vi "Error Handle.vi"() -> ()   [LabVIEW 2016]
uses:
  <vilib>/Utility/error.llb/DialogType.ctl
  Architecture/Queue Management/ARC_Queue Create_Single.vi
  Architecture/Queue Management/ARC_Queue Valid.vi
  Architecture/Queue Management/ARC_Queue Insert Element.vi
  Architecture/Queue Management/ARC_Queue Remove Element.vi
  Architecture/Queue Management/ARC_Queue Destroy_Single.vi
panel:
  in  "Parameter":cluster{"Q-Local":string, "Variant":variant}
  out "Error Report":string
  out "Current State":string
  in  "Exit Program":bool
  in  "TempVariable":T1
  # "/* -------- Notes for All Users -------- */\nRecommand : \n[1].Display Setting Resolution -> 1440x900\n[2].Read Arch Notes First.\n[3].Make A Call When You Are In Trouble.\n\nTeam Members:\nPansino Soft,Pansino SDMA\n\nCopyright@2013 Pansino.Beijing\n\nVersion Number: 2013"
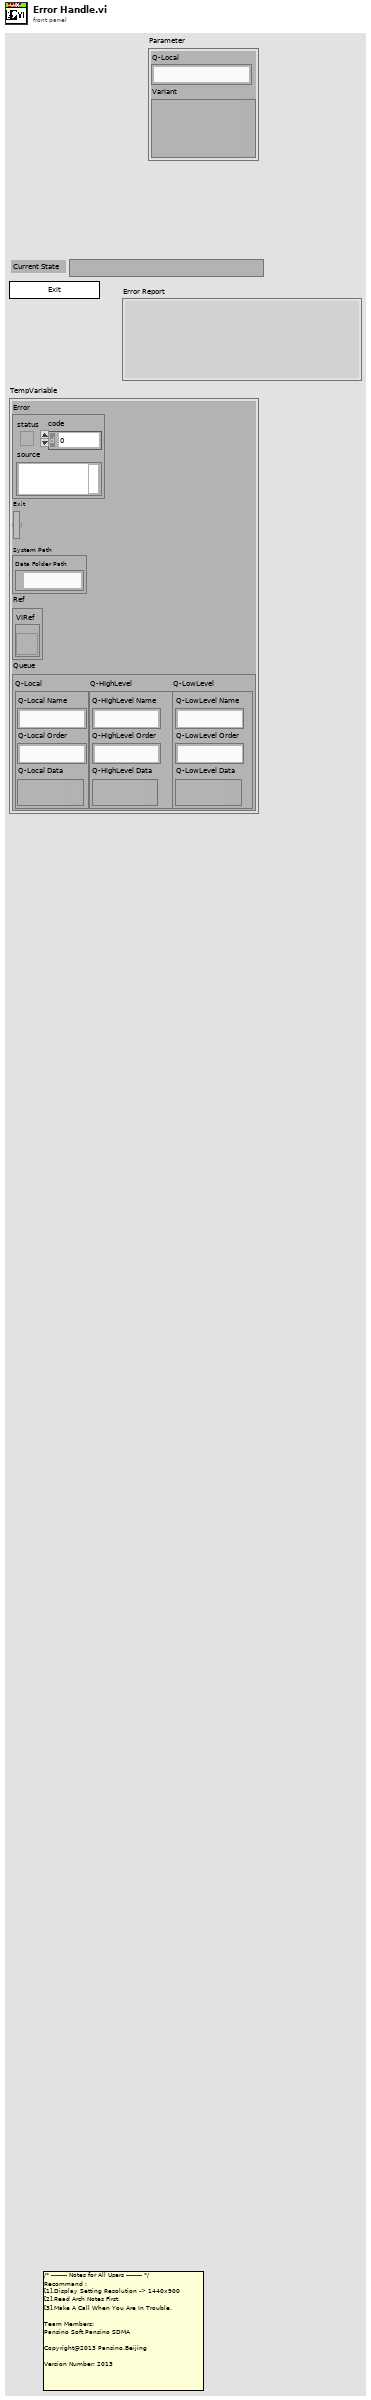
[diagram p1: front panel]
types:
  T1 = cluster{"Error":errorcluster, "Exit":bool, "System Path":cluster{"Data Folder Path":path}, "Ref":cluster{"VIRef":refnum<vi>}, "Queue":cluster{"Q-Local":cluster{"Q-Local Name":string, "Q-Local Order":string, "Q-Local Data":variant}, "Q-HighLevel":cluster{"Q-HighLevel Name":string, "Q-HighLevel Order":string, "Q-HighLevel Data":variant}, "Q-LowLevel":cluster{"Q-LowLevel Name":string, "Q-LowLevel Order":string, "Q-LowLevel Data":variant}}}
  T2 = typedef "DialogType.ctl" = u16
  T3 = cluster{"DfltDataFolder":path, "ParaFolder":path, "SysCfg":path, "CHdef":path, "ModCfg":path, "DT Folder":path, "ErrorLog":path, "HBMlic":path, "HBMDriver":path}
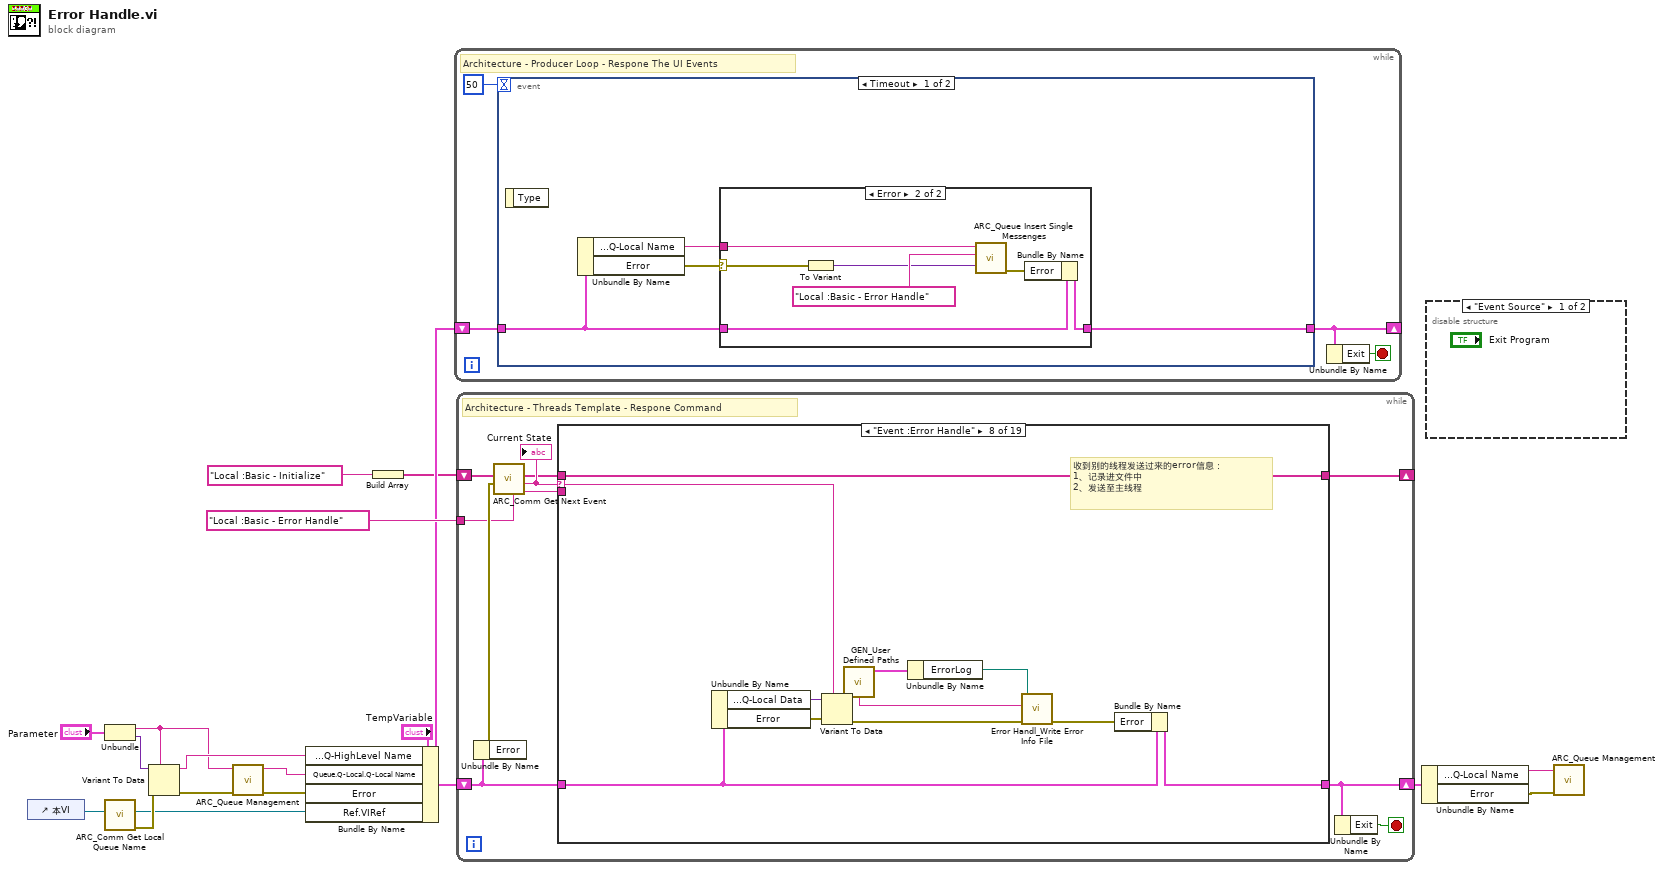
[diagram p0: block diagram]
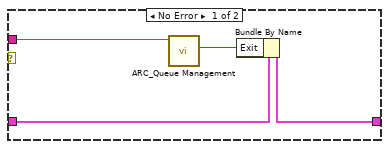
[diagram p2: hidden frame]
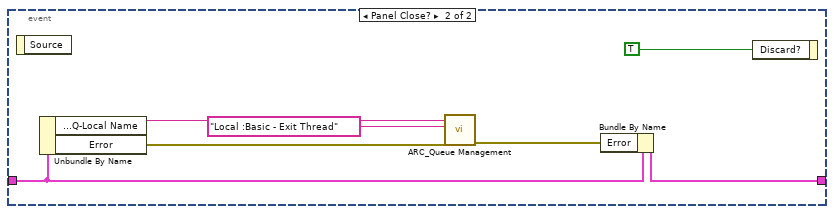
[diagram p3: hidden frame]
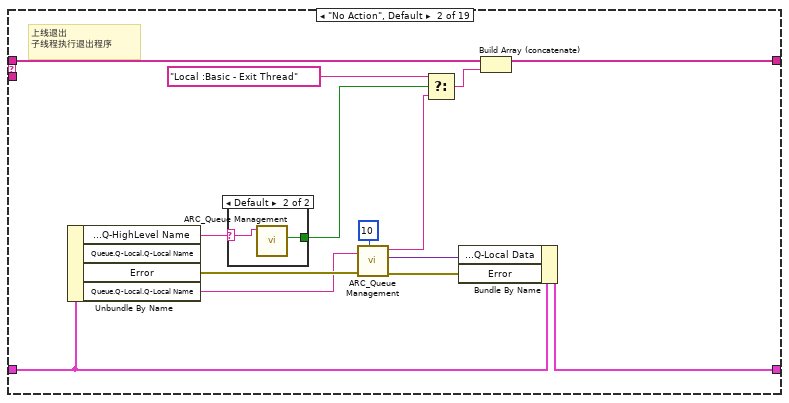
[diagram p6: hidden frame]
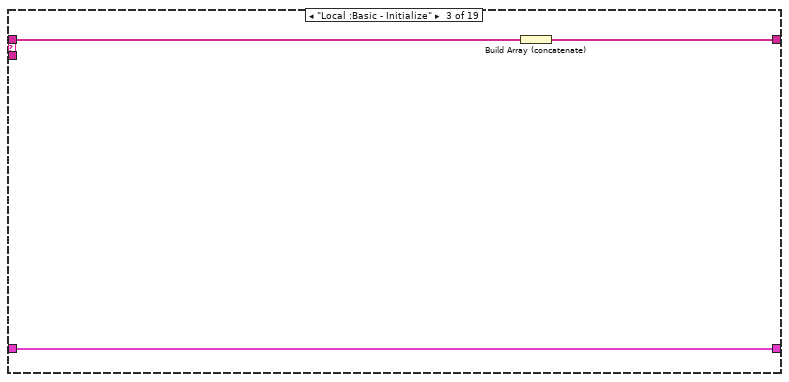
[diagram p8: hidden frame]
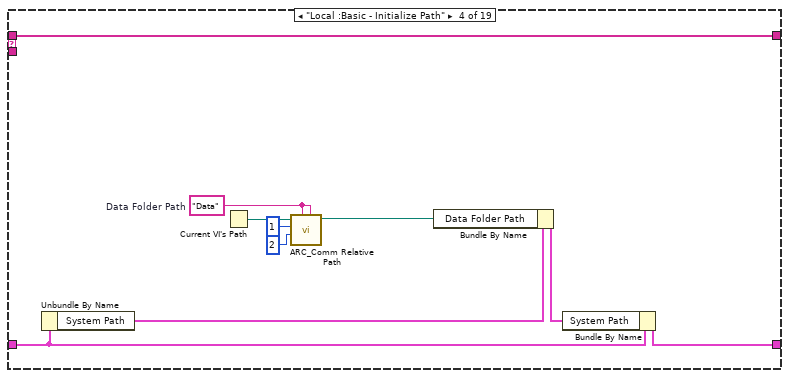
[diagram p9: hidden frame]
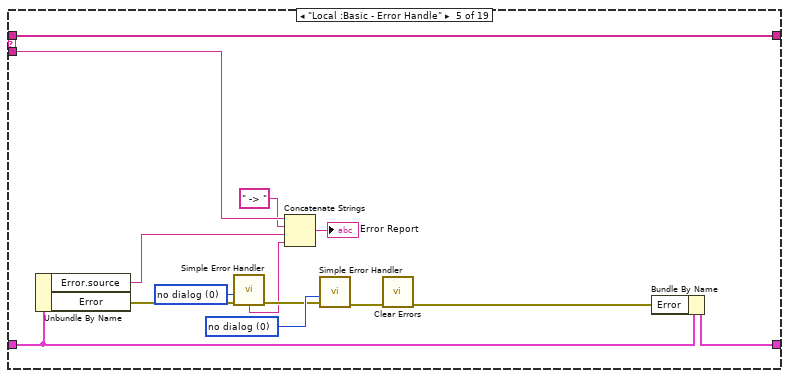
[diagram p10: hidden frame]
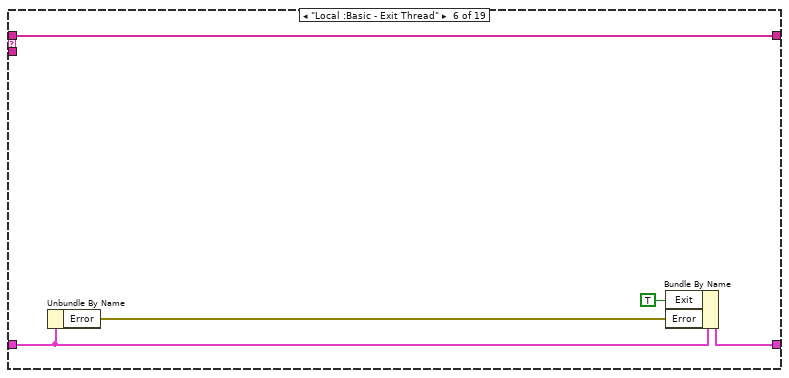
[diagram p11: hidden frame]
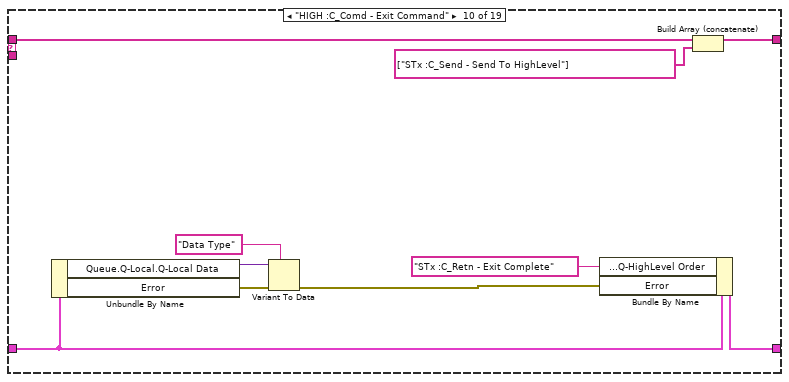
[diagram p14: hidden frame]
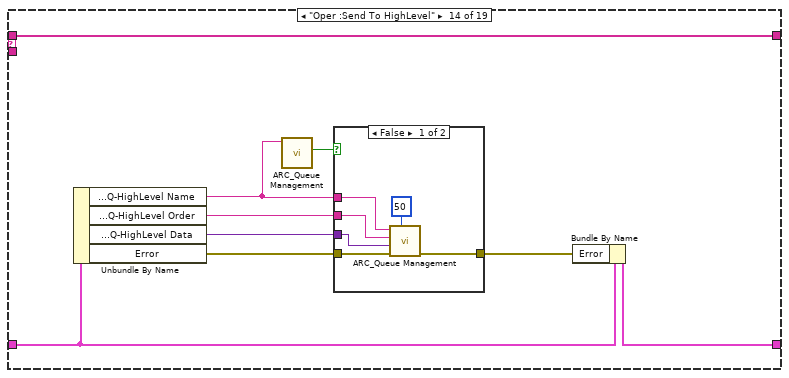
[diagram p18: hidden frame]
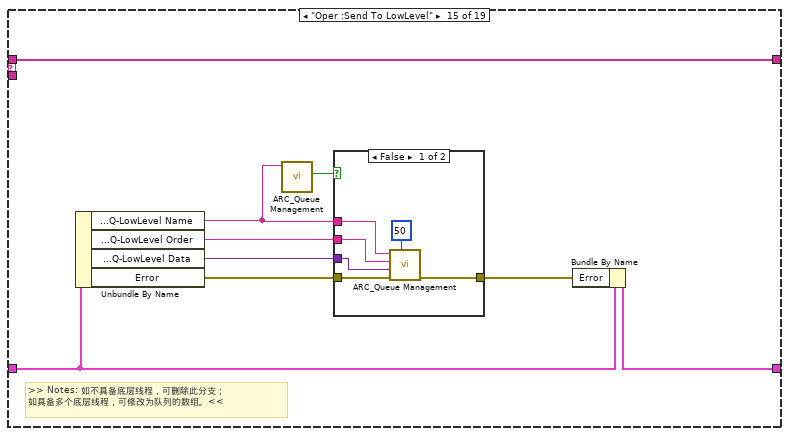
[diagram p20: hidden frame]
diagram:
  n1 = control-ref of="本VI"() -> (w7:refnum<vi>)
  n2 = Unbundle("Parameter") -> ("Q-Local"=w1:string, "Variant"=w10:variant)
  n3 = call "ARC_Comm Get Local Queue Name.vi"("VI Ref"=w7) -> ("error out"=w8:errorcluster, "VI Ref out"=w5:refnum<vi>)  [unwired: 8 in, 1 out]
  n4 = Variant To Data(error in=w8, type=w1, Variant=w10) -> (data=w2:string, error out=w6:errorcluster)
  n5 = call-poly "ARC_Queue Management.vi"("error in"=w6, "Queue Name"=w1) -> ("error out"=w4:errorcluster, "Queue Name dup"=w3:string)  [unwired: 7 in, 1 out]
  n6 = Bundle By Name(cluster="TempVariable", "Queue.Q-HighLevel.Q-HighLevel Name"=w2, "Queue.Q-Local.Q-Local Name"=w3, "Error"=w4, "Ref.VIRef"=w5) -> (w13:T1)
  n7 = Build Array("Local :Basic - Initialize") -> (w11:string[])
  n8 = while {
    shift-right: [w20] -> _
    shift-left: w13 -> [w21]
    stop <- w19 stop-if-true
    # "Architecture - Producer Loop - Respone The UI Events"
    n9 = event shown="[0] Timeout" {
      selector: _ -> [_ _]
      dyn-events: _ -> [_ _]
      timeout: 50 -> [_ _]
      tunnel: w21 -> [w25 w42]
      tunnel: [w26 w41] -> w20
      event Timeout {
        n10 = event-data() -> ()  [unwired: 1 in, 1 out]
        n11 = Unbundle By Name(w25) -> ("Queue.Q-Local.Q-Local Name"=w24:string, "Error"=w23:errorcluster)
        n12 = case shown="Error" w23 {
          selector: w23 -> [_ w37]
          tunnel: [w30 w35] -> w26
          tunnel: w25 -> [w28 w36]
          tunnel: w24 -> [w27 w34]
          frame No Error {
            n13 = call-poly "ARC_Queue Management.vi"("Queue Name(unamed)"=w27) -> ("Not Exist?"=w29:bool)  [unwired: 8 in, 2 out]
            n14 = Bundle By Name(cluster=w28, "Exit"=w29) -> (w30:T1)
          }
          frame Error {
            n15 = To Variant(anything=w37) -> (Variant=w32:variant)
            n16 = call "ARC_Queue Insert Single Messenges.vi"("Data"=w32, "Order"="Local :Basic - Error Handle" ("Event"), "Queue Name"=w34) -> ("error out"=w31:errorcluster)  [unwired: 8 in]
            n17 = Bundle By Name(cluster=w36, "Error"=w31) -> (w35:T1)
          }
        }
      }
      event Panel Close? {
        n18 = event-data() -> ()  [unwired: 1 in, 1 out]
        n19 = Unbundle By Name(w42) -> ("Queue.Q-Local.Q-Local Name"=w39:string, "Error"=w43:errorcluster)
        n20 = call-poly "ARC_Queue Management.vi"("error in (no error)"=w43, "Event"="Local :Basic - Exit Thread", "Queue Name(unamed)"=w39) -> ("error out"=w40:errorcluster)  [unwired: 7 in, 1 out]
        n21 = Bundle By Name(cluster=w42, "Error"=w40) -> (w41:T1)
        n22 = event-data("Discard?"=TRUE ("放弃？")) -> ()  [unwired: 1 in, 1 out]
      }
    }
    n23 = Unbundle By Name(w20) -> ("Exit"=w19:bool)
  }
  n24 = while {
    shift-right: [w48] -> w18
    shift-left: w13 -> [w50]
    shift-right: [w51] -> _
    shift-left: w11 -> [w54]
    tunnel: "Local :Basic - Error Handle" ("Error Handle") -> [w46]
    stop <- w47 stop-if-true
    # "Architecture - Threads Template - Respone Command"
    n25 = Unbundle By Name(w50) -> ("Error"=w49:errorcluster)
    n26 = call "ARC_Comm Get Next Event.vi"("Error Handle"=w46, "error in (no error)"=w49, "event queue in"=w54) -> ("prev event"=w45:string, "next event"=w53:string, "event queue out"=w52:string[])  [unwired: 3 in]
    "Current State" <- w53
    n27 = case shown="\"Event :Error Handle\"" w53 {
      selector: w53 -> [_ _ _ _ _ _ _ w113 _ _ _ _ _ _ _ _ _ _ _]
      tunnel: w50 -> [w55 w70 w74 w83 w97 w101 w105 w116 w118 w126 w130 w132 w134 w141 w157 w168 w173 w180 w186]
      tunnel: w52 -> [w56 w63 w75 w85 w99 w104 w106 w117 w119 w129 w131 w133 w135 w144 w160 w169 w171 w181 w184]
      tunnel: [w56 w62 w73 w85 w99 w104 w106 w117 w119 w127 w131 w133 w135 w144 w160 w169 w170 w181 w183] -> w51
      tunnel: [w55 w69 w74 w84 w98 w102 w105 w108 w118 w128 w130 w132 w134 w140 w156 w168 w172 w179 w185] -> w48
      tunnel: w45 -> [_ _ _ _ w90 _ _ _ _ _ _ _ _ _ _ _ _ _ _]
      frame "----------Core Status----------" {
      }
      frame "No Action", Default {
        # "上线退出\n子线程执行退出程序"
        n28 = Unbundle By Name(w70) -> ("Queue.Q-HighLevel.Q-HighLevel Name"=w65:string, "Error"=w66:errorcluster, "Queue.Q-Local.Q-Local Name"=w64:string)  [unwired: 1 out]
        n29 = case shown="Default" w65 {
          selector: w65 -> [_ w71]
          tunnel: [_ w72] -> w60
          frame "" {
          }
          frame Default {
            n30 = call-poly "ARC_Queue Management.vi"("Queue Name(unamed)"=w71) -> ("Not Exist?"=w72:bool)  [unwired: 8 in, 2 out]
          }
        }
        n31 = call-poly "ARC_Queue Management.vi"("Time out(-1)_queue out"=10, "error in (no error)"=w66, "Queue Name(unamed)"=w64) -> ("error out"=w68:errorcluster, "Data"=w67:variant, "Event"=w58:string)  [unwired: 5 in, 1 out]
        n32 = Select(t="Local :Basic - Exit Thread" ("Event"), s=w60, f=w58) -> (s? t:f=w57:string)
        n33 = Bundle By Name(cluster=w70, "Queue.Q-Local.Q-Local Data"=w67, "Error"=w68) -> (w69:T1)
        n34 = Build Array (concatenate)(w63, w57) -> (w62:string[])
      }
      frame "Local :Basic - Initialize" {
        n35 = Build Array (concatenate)(w75) -> (w73:string[])
      }
      frame "Local :Basic - Initialize Path" {
        w78 = "Data"  # Data Folder Path
        n36 = Unbundle By Name(w83) -> ("System Path"=w77:cluster{"Data Folder Path":path})
        n37 = Current VI's Path() -> (path=w79:path)
        n38 = call "ARC_Comm Relative Path.vi"("Development Relative Path"=w78, "Run Time relative path"=w78, "Run-Time File Depth"=2, "Development File Depth"=1, "Root Path"=w79) -> ("Relative Path"=w82:path)  [unwired: 5 in, 1 out]
        n39 = Bundle By Name(cluster=w77, "Data Folder Path"=w82) -> (w76:cluster{"Data Folder Path":path})
        n40 = Bundle By Name(cluster=w83, "System Path"=w76) -> (w84:T1)
      }
      frame "Local :Basic - Error Handle" {
        w91 = T2 0 items=["no dialog", "OK message", "continue or stop message", "OK message + warnings", "continue/stop + warnings"] ("type of dialog (OK msg:1)")
        w94 = T2 0 items=["no dialog", "OK message", "continue or stop message", "OK message + warnings", "continue/stop + warnings"] ("type of dialog (OK msg:1)")
        n41 = Unbundle By Name(w97) -> ("Error.source"=w86:string, "Error"=w93:errorcluster)
        n42 = call <vilib>:"Simple Error Handler.vi"("type of dialog (OK msg:1)"=w91, "error in (no error)"=w93) -> ("error out"=w92:errorcluster, "message"=w88:string)  [unwired: 3 in, 3 out]
        n43 = Concatenate Strings(w90, " -> " ("字符串"), w86, w88) -> (→"Error Report":string)
        n44 = call <vilib>:"Simple Error Handler.vi"("type of dialog (OK msg:1)"=w94, "error in (no error)"=w92) -> ("error out"=w96:errorcluster)  [unwired: 3 in, 4 out]
        n45 = call <vilib>:"Clear Errors.vi"("error in (no error)"=w96) -> ("error out"=w95:errorcluster)  [unwired: 5 in, 1 out]
        n46 = Bundle By Name(cluster=w97, "Error"=w95) -> (w98:T1)
      }
      frame "Local :Basic - Exit Thread" {
        n47 = Unbundle By Name(w101) -> ("Error"=w103:errorcluster)
        n48 = Bundle By Name(cluster=w101, "Exit"=TRUE, "Error"=w103) -> (w102:T1)
      }
      frame "----------------Events--------------" {
      }
      frame "Event :Error Handle" {
        # "收到别的线程发送过来的error信息：\n1、记录进文件中\n2、发送至主线程"
        n49 = Unbundle By Name(w116) -> ("Queue.Q-Local.Q-Local Data"=w114:variant, "Error"=w115:errorcluster)
        n50 = Variant To Data(error in=w115, type=w113, Variant=w114) -> (data=w111:string, error out=w112:errorcluster)
        n51 = call "GEN_User Defined Paths.vi"() -> ("UserDefinedPath"=w110:T3)  [unwired: 11 in]
        n52 = Unbundle By Name(w110) -> ("ErrorLog"=w109:path)
        n53 = call "Error Handl_Write Error Info File.vi"("error in"=w112, "Error Info"=w111, "Error log file"=w109) -> ("error out"=w107:errorcluster)  [unwired: 8 in]
        n54 = Bundle By Name(cluster=w116, "Error"=w107) -> (w108:T1)
      }
      frame "----------Commond From HIGH----------" {
      }
      frame "HIGH :C_Comd - Exit Command" {
        n55 = Unbundle By Name(w126) -> ("Queue.Q-Local.Q-Local Data"=w125:variant, "Error"=w124:errorcluster)
        n56 = Variant To Data(error in=w124, type="Data Type" ("Data Type"), Variant=w125) -> (error out=w122:errorcluster)  [unwired: 1 out]
        n57 = Bundle By Name(cluster=w126, "Queue.Q-HighLevel.Q-HighLevel Order"="STx :C_Retn - Exit Complete" ("Data Type"), "Error"=w122) -> (w128:T1)
        n58 = Build Array (concatenate)(w129, string[] ["STx :C_Send - Send To HighLevel"] ("数组")) -> (w127:string[])
      }
      frame "----------Operation----------" {
      }
      frame "Oper :" {
      }
      frame "----------Communication----------" {
      }
      frame "Oper :Send To HighLevel" {
        n59 = Unbundle By Name(w141) -> ("Queue.Q-HighLevel.Q-HighLevel Name"=w143:string, "Queue.Q-HighLevel.Q-HighLevel Order"=w138:string, "Queue.Q-HighLevel.Q-HighLevel Data"=w137:variant, "Error"=w142:errorcluster)
        n60 = call-poly "ARC_Queue Management.vi"("Queue Name(unamed)"=w143) -> ("Not Exist?"=w139:bool)  [unwired: 8 in, 2 out]
        n61 = case shown="False" w139 {
          tunnel: w142 -> [w150 w151]
          tunnel: w143 -> [w148 _]
          tunnel: w138 -> [w146 _]
          tunnel: w137 -> [w147 _]
          tunnel: [w145 w151] -> w136
          frame False {
            n62 = call-poly "ARC_Queue Management.vi"("Time out(-1)_queue in"=50, "error in (no error)"=w150, "Data"=w147, "Event"=w146, "Queue Name(unamed)"=w148) -> ("error out"=w145:errorcluster)  [unwired: 5 in, 1 out]
          }
          frame True {
          }
        }
        n63 = Bundle By Name(cluster=w141, "Error"=w136) -> (w140:T1)
      }
      frame "Oper :Send To LowLevel" {
        # ">> Notes: 如不具备底层线程，可删除此分支；\n如具备多个底层线程，可修改为队列的数组。<<"
        n64 = Unbundle By Name(w157) -> ("Queue.Q-LowLevel.Q-LowLevel Name"=w159:string, "Queue.Q-LowLevel.Q-LowLevel Order"=w154:string, "Queue.Q-LowLevel.Q-LowLevel Data"=w153:variant, "Error"=w158:errorcluster)
        n65 = call-poly "ARC_Queue Management.vi"("Queue Name(unamed)"=w159) -> ("Not Exist?"=w155:bool)  [unwired: 8 in, 2 out]
        n66 = case shown="False" w155 {
          tunnel: w158 -> [w166 w167]
          tunnel: w159 -> [w164 _]
          tunnel: w154 -> [w162 _]
          tunnel: w153 -> [w163 _]
          tunnel: [w161 w167] -> w152
          frame False {
            n67 = call-poly "ARC_Queue Management.vi"("Time out(-1)_queue in"=50, "error in (no error)"=w166, "Data"=w163, "Event"=w162, "Queue Name(unamed)"=w164) -> ("error out"=w161:errorcluster)  [unwired: 5 in, 1 out]
          }
          frame True {
          }
        }
        n68 = Bundle By Name(cluster=w157, "Error"=w152) -> (w156:T1)
      }
      frame "----------Respond From LOW----------" {
      }
      frame "LOW :C_Resp - /* ADD NAME */" {
        n69 = Unbundle By Name(w173) -> ("Error"=w174:errorcluster)
        n70 = Build Array (concatenate)(w171) -> (w170:string[])
        n71 = Bundle By Name(cluster=w173, "Error"=w174) -> (w172:T1)
      }
      frame "LOW :C_Resp - /*Respond The Request*/" {
        n72 = Unbundle By Name(w180) -> ("Queue.Q-Local.Q-Local Data"=w177:variant, "Error"=w178:errorcluster)
        n73 = Variant To Data(error in=w178, type="Data Type" ("Data Type"), Variant=w177) -> (error out=w176:errorcluster)  [unwired: 1 out]
        n74 = Bundle By Name(cluster=w180, "Error"=w176) -> (w179:T1)
      }
      frame "LOW :C_Resp - Exit Complete" {
        # ">> Notes: 此处接收下层的返回指令；: 前代表下层的VI功能名，如ACTS等<<"
        n75 = Unbundle By Name(w186) -> ("Error"=w187:errorcluster)
        n76 = Build Array (concatenate)(w184, string[] ["STx :L_Core - Exit Thread"] ("数组")) -> (w183:string[])
        n77 = Bundle By Name(cluster=w186, "Error"=w187) -> (w185:T1)
      }
    }
    n78 = Unbundle By Name(w48) -> ("Exit"=w47:bool)
  }
  n79 = Unbundle By Name(w18) -> ("Queue.Q-Local.Q-Local Name"=w16:string, "Error"=w17:errorcluster)
  n80 = disable-structure shown="\"Event Source\"" {
    frame condition #0 (active) {
    }
    frame condition #1 {
    }
  }
  n81 = call-poly "ARC_Queue Management.vi"("error in (no error)"=w17, "Queue Name(unamed)"=w16) -> ()  [unwired: 7 in, 3 out]
